vi "Write VacuumLine Params.vi"(8 "error in (no error)":errorcluster, 10 "Position Params":T1 {"max( |Motor Pos - LRF Distance| )" min=0.0}, 11 "VacuumLine in":refnum<class "VacuumLine.lvclass">) -> (0 "error out":errorcluster, 3 "VacuumLine out":refnum<class "VacuumLine.lvclass">)   [LabVIEW 2016, in "Hardware.lvlib" / "VacuumLine.lvlib" / "VacuumLine.lvclass"]
uses:
  <userlib>/Common Components/Hardware/Abstract System/VacuumLine/VacuumLine/VacuumLine.lvclass
  <userlib>/Common Components/Hardware/Abstract System/VacuumLine/VacuumLine/VacuumLine Params.ctl
  <userlib>/Common Components/Hardware/Abstract System/VacuumLine/VacuumLine/Valve Complex.ctl
  <userlib>/Common Components/Hardware/Abstract System/VacuumLine/VacuumLine/Logic Cluster.ctl
  <userlib>/Common Components/Hardware/Abstract System/VacuumLine/VacuumLine/VacuumLine.lvclass/VacuumLine.ctl
panel:
  # "Pin#"
  # "Location"
  # "Tolerance"
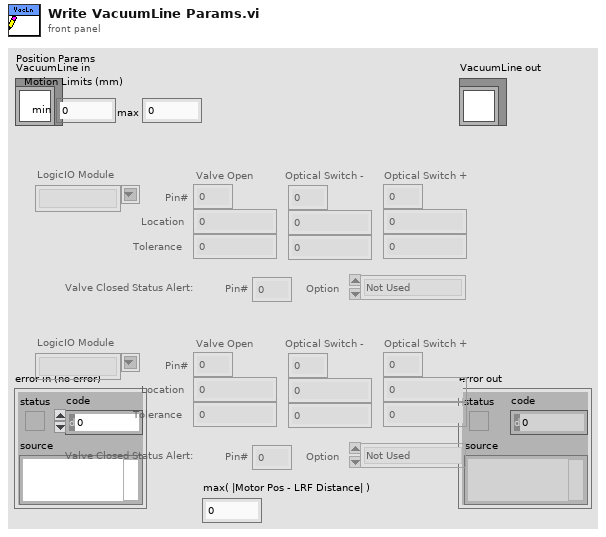
[diagram p1: front panel]
types:
  T1 = typedef "Hardware.lvlib/VacuumLine.lvlib/VacuumLine.lvclass/VacuumLine Params.ctl" = cluster{"Motion Limits":cluster{"min":dbl, "max":dbl}, "Valve Complexes":T2[], "max( |Motor Pos - LRF Distance| )":dbl}
  T2 = typedef "Hardware.lvlib/VacuumLine.lvlib/VacuumLine.lvclass/Valve Complex.ctl" = cluster{"LogicIO Module":string, "Valve Open":T3, "Optical Switch -":T3, "Optical Switch +":T3, "Valve Closed Status Alert":cluster{"Pin#":u8, "Option":enum16{"Not Used", "Normally Closed"}}}
  T3 = typedef "Hardware.lvlib/VacuumLine.lvlib/VacuumLine.lvclass/Logic Cluster.ctl" = cluster{"Pin#":u8, "Location":dbl, "Tolerance":dbl}
  T4 = cluster{"valve":bool, "optical switch -":bool, "optical switch +":bool, "Valve Closed Status Alert":bool}
  T5 = cluster{"valve":bool, "optical switch -":bool, "optical switch +":bool, "Valve Closed Status Alert":bool}[]
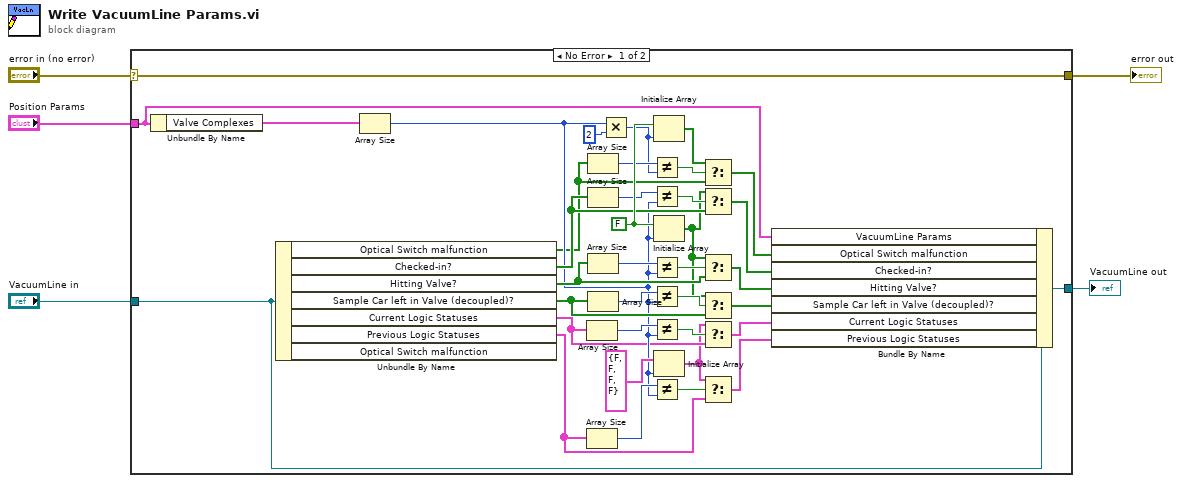
[diagram p0: block diagram]
diagram:
  n1 = case shown="No Error" "error in (no error)" {
    selector: "error in (no error)" -> [w42 w43]
    tunnel: [w42 w43] -> w4
    tunnel: [w41 w44] -> w2
    tunnel: "VacuumLine in" -> [w35 w44]
    tunnel: "Position Params" -> [w40 _]
    frame No Error {
      w39 = FALSE
      n2 = Unbundle By Name(w40) -> ("Valve Complexes"=w38:T2[])
      n3 = Unbundle By Name(w35) -> ("Optical Switch malfunction"=w7:bool[], "Checked-in?"=w32:bool[], "Hitting Valve?"=w24:bool[], "Sample Car left in Valve (decoupled)?"=w20:bool[], "Current Logic Statuses"=w12:T5, "Previous Logic Statuses"=w11:T5)  [unwired: 1 out]
      n4 = Array Size(array=w38) -> (size(s)=w13:i32)
      n5 = Array Size(array=w12) -> (size(s)=w17:i32)
      n6 = Array Size(array=w11) -> (size(s)=w16:i32)
      n7 = Array Size(array=w7) -> (size(s)=w18:i32)
      n8 = Array Size(array=w32) -> (size(s)=w34:i32)
      n9 = Array Size(array=w24) -> (size(s)=w30:i32)
      n10 = Array Size(array=w20) -> (size(s)=w22:i32)
      n11 = Multiply(x=w13, y=2 ("x")) -> (x*y=w15:i32)
      n12 = Not Equal?(x=w18, y=w15) -> (x != y?=w27:bool)
      n13 = Not Equal?(x=w34, y=w13) -> (x != y?=w33:bool)
      n14 = Not Equal?(x=w30, y=w13) -> (x != y?=w29:bool)
      n15 = Not Equal?(x=w22, y=w13) -> (x != y?=w28:bool)
      n16 = Not Equal?(x=w17, y=w13) -> (x != y?=w26:bool)
      n17 = Not Equal?(x=w16, y=w13) -> (x != y?=w25:bool)
      n18 = Initialize Array(w39, w15) -> (w14:bool[])
      n19 = Initialize Array(w39, w13) -> (w21:bool[])
      n20 = Initialize Array(T4 {"valve"=FALSE, "optical switch -"=FALSE, "optical switch +"=FALSE, "Valve Closed Status Alert"=FALSE} ("Cluster"), w13) -> (w10:T5)
      n21 = Select(t=w14, s=w27, f=w7) -> (s? t:f=w6:bool[])
      n22 = Select(t=w21, s=w33, f=w32) -> (s? t:f=w31:bool[])
      n23 = Select(t=w21, s=w29, f=w24) -> (s? t:f=w23:bool[])
      n24 = Select(t=w21, s=w28, f=w20) -> (s? t:f=w19:bool[])
      n25 = Select(t=w10, s=w26, f=w12) -> (s? t:f=w9:T5)
      n26 = Select(t=w10, s=w25, f=w11) -> (s? t:f=w8:T5)
      n27 = Bundle By Name(cluster=w35, "VacuumLine Params"=w40, "Optical Switch malfunction"=w6, "Checked-in?"=w31, "Hitting Valve?"=w23, "Sample Car left in Valve (decoupled)?"=w19, "Current Logic Statuses"=w9, "Previous Logic Statuses"=w8) -> (w41:refnum<class "VacuumLine.lvclass">)
    }
    frame Error {
    }
  }
  "error out" <- w4
  "VacuumLine out" <- w2
